vi "FPGA_GetRef.vi"(2 "error in (no error)":errorcluster) -> (0 "error out":errorcluster, 1 "FPGA_Ref":refnum<k20>)   [LabVIEW 2009, in "FPGA.lvlib"]
uses:
  FPGA.lvlib
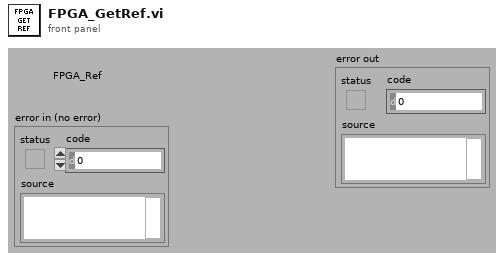
[diagram p1: front panel]
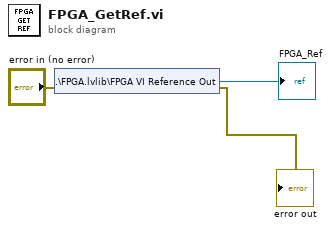
[diagram p0: block diagram]
diagram:
  n1 = shared-variable ".\\FPGA.lvlib\\FPGA VI Reference Out"(error in="error in (no error)") -> (→"FPGA_Ref":refnum<k20>, error out=→"error out":errorcluster)
